vi "MS SQL_Read_STN_Count_machine_code.vi"(8 "error in (no error)":errorcluster, 9 "Table?":string, 10 "Query":string, 11 "Refnum in":T1) -> (0 "error out":errorcluster, 1 "MACHINECODE":string[](array[string]), 2 "Count":i64, 3 "Refnum out":T1)   [LabVIEW 2020]
uses:
  <vilib>/addons/database/Connection.llb/Conn ObjectReference.ctl
  <vilib>/addons/database/NI_Database_API.lvlib
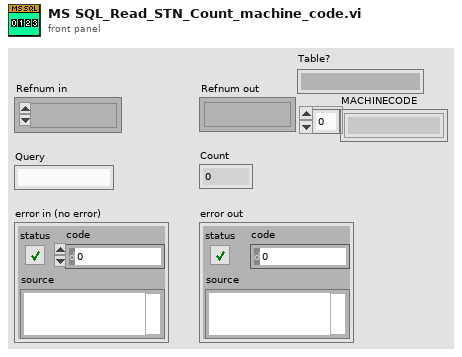
[diagram p1: front panel]
types:
  T1 = typedef "NI_Database_API.lvlib/Conn ObjectReference.ctl" = refnum<k1>
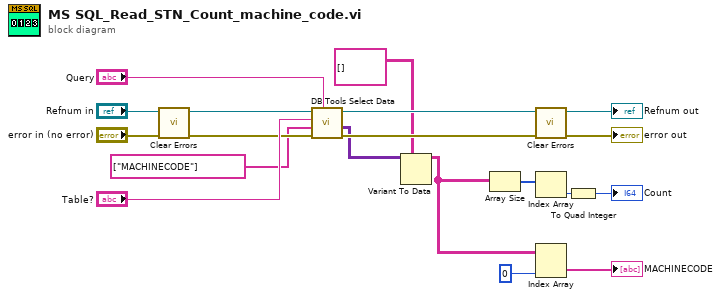
[diagram p0: block diagram]
diagram:
  n1 = call <vilib>:"Clear Errors.vi"("error in (no error)"="error in (no error)") -> ("error out"=w4:errorcluster)  [unwired: 5 in, 1 out]
  n2 = call <vilib>:"DB Tools Select Data.vi"("condition"="Query", "error in (no error)"=w4, "columns"=string[] ["MACHINECODE"], "table"="Table?", "connection reference"="Refnum in") -> ("error out"=w13:errorcluster, "data"=w2:variant[][], "connection reference out"=→"Refnum out":T1)  [unwired: 1 in]
  n3 = Variant To Data(type=string[][] [] ("Data"), Variant=w2) -> (data=w7:string[][])  [unwired: 1 in, 1 out]
  n4 = Array Size(array=w7) -> (size(s)=w11:i32[])
  n5 = call <vilib>:"Clear Errors.vi"("error in (no error)"=w13) -> ("error out"=→"error out":errorcluster)  [unwired: 5 in, 1 out]
  n6 = Index Array(array=w11) -> (element=w10:i32)  [unwired: 1 in]
  n7 = Index Array(array=w7, index (col)=0 ("disabled index (col)")) -> (element=→"MACHINECODE":string[])  [unwired: 1 in]
  n8 = To Quad Integer(1:w10) -> (0:→"Count":i64)
